vi "OldClimbGetSensorPoseLeft.vi"() -> (1 "ClimbGetSensorPoseLeft":dbl)   [LabVIEW 2023]
uses:
  OldClimbGlobal.vi
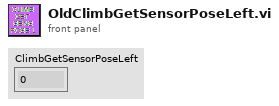
[diagram p1: front panel]
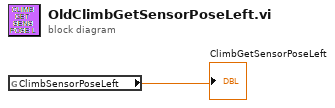
[diagram p0: block diagram]
diagram:
  n1 = global read "OldClimbGlobal.vi" "ClimbSensorPoseLeft"() -> (→"ClimbGetSensorPoseLeft":dbl)
